vi "demo_GDevCon Global Explosion.vi"(11 "Stop Demo":refnum<user-event>) -> ()   [LabVIEW 2020]
panel:
  # "GDevCon is an independent conference open to all graphical developers\n\nOrganised by leaders in the LabVIEW™ community, GDevCon is focused on delivering world-class graphical programming material covering a wide spread of topics relevant to today’s discerning developer.\nhttps://gdevcon.com/\nhttps://gdevcon.com/spin-offs/"
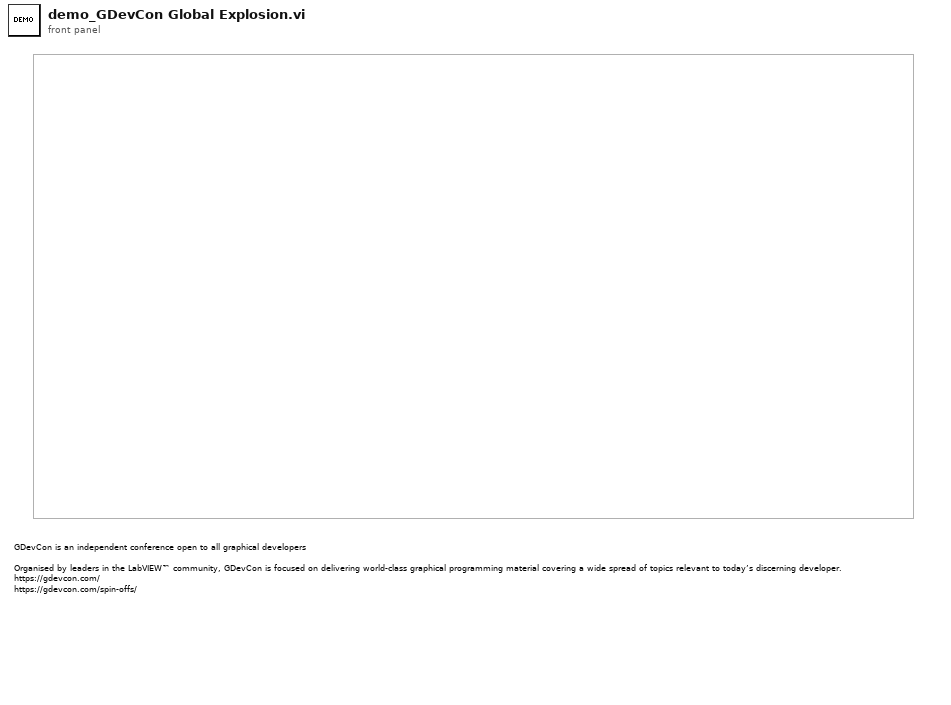
[diagram p1: front panel]
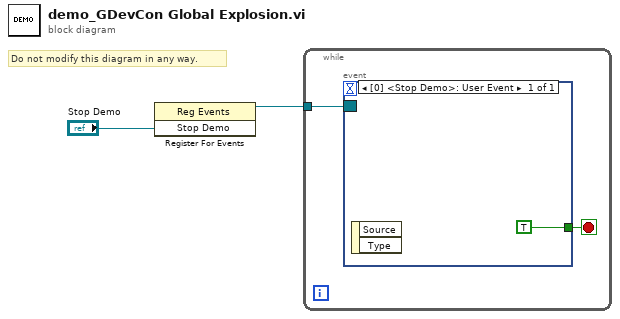
[diagram p0: block diagram]
diagram:
  # "Do not modify this diagram in any way."
  n1 = register-events("Stop Demo") -> (reference out=w1:refnum<event-registration>)  [unwired: 2 in, 1 out]
  n2 = while {
    tunnel: w1 -> [w4]
    stop <- w3 stop-if-true
    n3 = event shown="[0] <Stop Demo>: User Event" {
      selector: w4 -> [_]
      dyn-events: _ -> [_]
      timeout: _ -> [_]
      tunnel: [TRUE] -> w3
      event User Event {
        n4 = event-data() -> ()  [unwired: 1 in, 2 out]
      }
    }
  }
